vi "Toggle.vi"(10 "Input":bool) -> (2 "Output":bool)   [LabVIEW 2014]
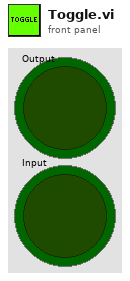
[diagram p1: front panel]
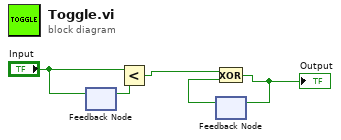
[diagram p0: block diagram]
diagram:
  n1 = feedback #1() -> (w5:bool)  [unwired: 1 in]
  n2 = feedback-in #1("Input") -> ()
  n3 = Less?(x="Input", y=w5) -> (x < y?=w4:bool)
  n4 = feedback #2() -> (w3:bool)  [unwired: 1 in]
  n5 = Exclusive Or(1:w3, 2:w4) -> (0:w1:bool)
  "Output" <- w1
  n6 = feedback-in #2(w1) -> ()
